vi "processOctaVolMatlab.vi"(0 "C2":dbl format="%#_13g", 3 "Output Path":path, 7 "C3":dbl format="%#_13g", 12 "Updated camera":T2, 14 "OCT filename out":string) -> ()   [LabVIEW 2017]
uses:
  <vilib>/vision/Image Controls.llb/IMAQ Image.ctl
  classes/HardwareObjects/Camera/Camera.lvclass
panel:
  in  "Camera in":refnum<class "Camera.lvclass">
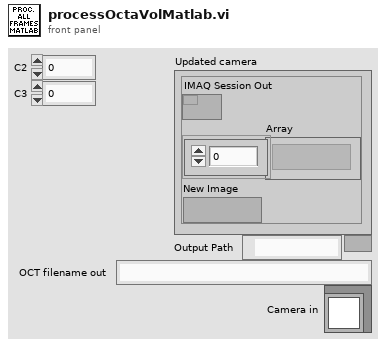
[diagram p1: front panel]
types:
  T1 = typedef "IMAQ Image.ctl" = refnum<image>
  T2 = cluster{"IMAQ Session Out":refnum<k11>, "Array":T1[], "New Image":T1}
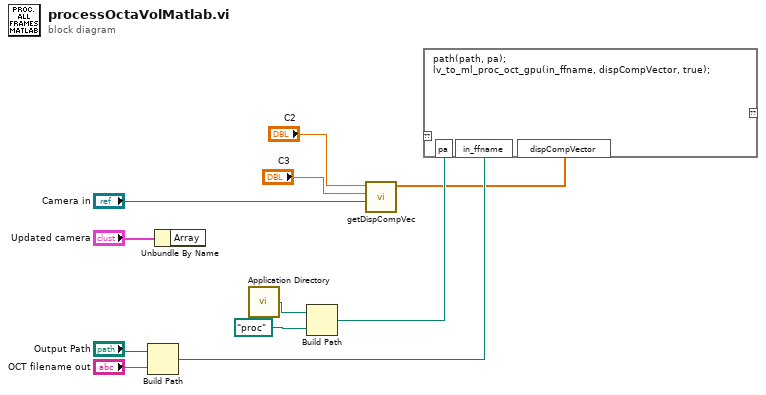
[diagram p0: block diagram]
diagram:
  n1 = Build Path(base path="Output Path", name or relative path="OCT filename out") -> (appended path=w8:path)
  n2 = Unbundle By Name("Updated camera") -> ()  [unwired: 1 out]
  n3 = call <vilib>:"Application Directory.vi"() -> ("Application Directory"=w7:path)
  n4 = Build Path(base path=w7, name or relative path=path "proc") -> (appended path=w4:path)
  n5 = call "getDispCompVec.vi"("Camera in"="Camera in", "C3"="C3", "C2"="C2") -> ("Gc"=w3:cdb[])  [unwired: 8 in]
  n6 = script code="path(path, pa);\nlv_to_ml_proc_oct_gpu(in_ffname, dispCompVector, true);"("pa"=w4, "in_ffname"=w8, "dispCompVector"=w3) -> ()  [unwired: 1 in, 1 out]
